vi "change directory permissions.vi"(0 "directory":path=path "C:/Program Files (x86)/National Instruments/RT Images/User Components", 5 "owner":T2={"read"=TRUE, "write"=TRUE, "execute"=TRUE}, 7 "group":T2={"read"=TRUE, "write"=TRUE, "execute"=TRUE}, 9 "others":T2={"read"=TRUE, "write"=TRUE, "execute"=TRUE}, 11 "error in":errorcluster, 12 "action (get)":T1) -> (4 "directory out":path, 6 "permissions":i16 format="%o", 15 "error out":errorcluster)   [LabVIEW 2016]
uses:
  file permissions action.ctl
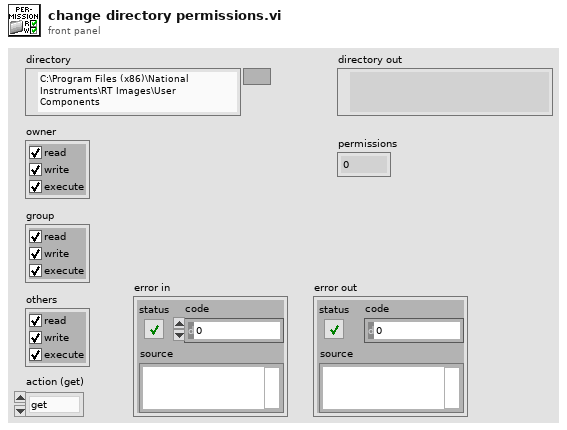
[diagram p1: front panel]
types:
  T1 = typedef "file permissions action.ctl" = enum16{"get", "set", "reset"}
  T2 = cluster{"read":bool, "write":bool, "execute":bool}
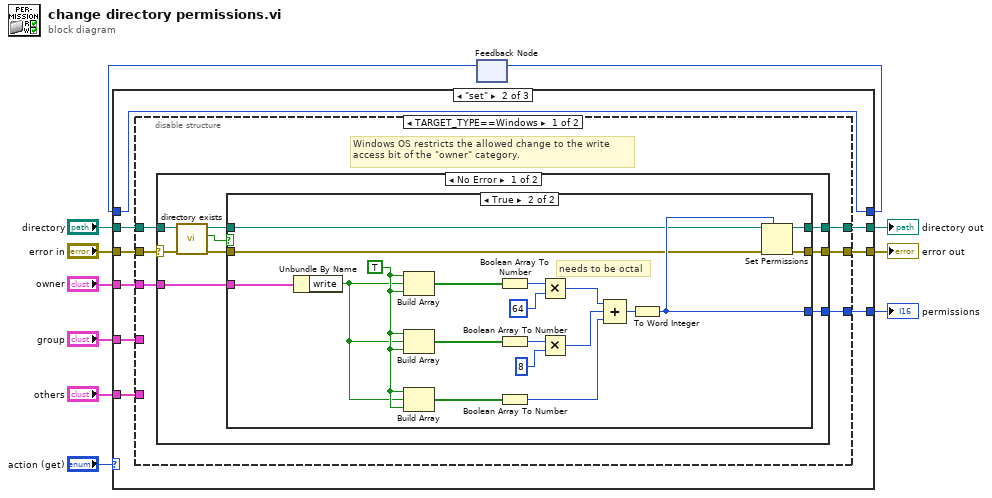
[diagram p0: block diagram]
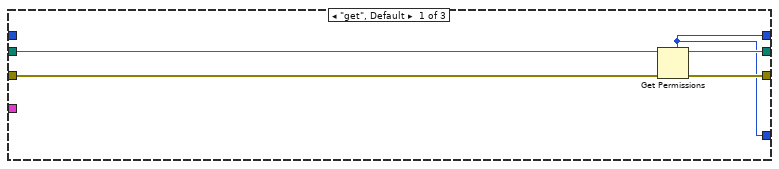
[diagram p2: hidden frame]
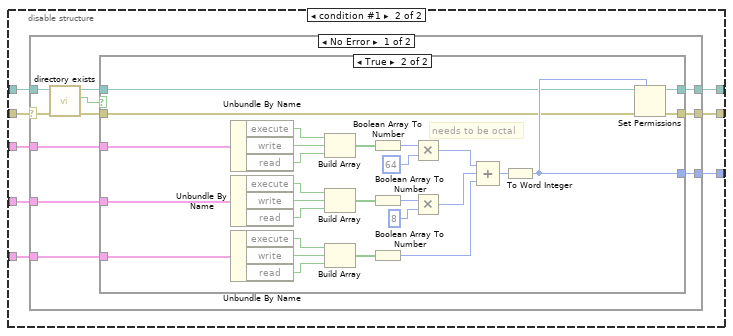
[diagram p5: hidden frame]
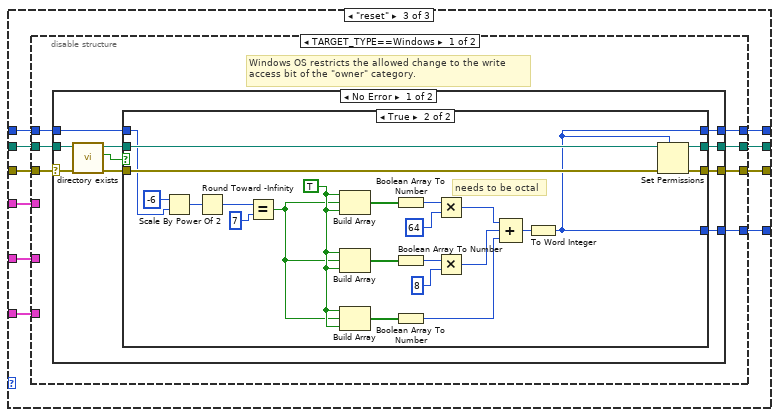
[diagram p8: hidden frame]
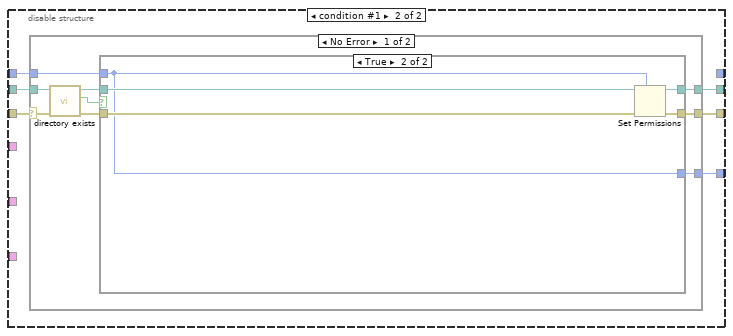
[diagram p11: hidden frame]
diagram:
  n1 = feedback #1() -> (w2:i16)  [unwired: 1 in]
  n2 = case shown="\"set\"" "action (get)" {
    tunnel: "directory" -> [w16 w25 w124]
    tunnel: "error in" -> [w15 w24 w123]
    tunnel: [w12 w17 w117] -> w3
    tunnel: w2 -> [_ w18 w116]
    tunnel: "owner" -> [_ w23 w122]
    tunnel: "group" -> [_ w22 w121]
    tunnel: "others" -> [_ w21 w120]
    tunnel: [w13 w20 w119] -> w4
    tunnel: [w14 w19 w118] -> w5
    tunnel: [w12 w18 w115] -> w1
    frame "get", Default {
      n3 = Get Permissions(8:w15, 11:w16) -> (0:w14:errorcluster, 3:w13:path, 5:w12:i16)  [unwired: 2 out]
    }
    frame "set" {
      n4 = disable-structure shown="TARGET_TYPE==Windows" {
        disable-tunnel: w25 -> [w31 w71]
        disable-tunnel: w24 -> [w26 w66]
        disable-tunnel: w23 -> [w30 w70]
        disable-tunnel: w22 -> [_ w65]
        disable-tunnel: w21 -> [_ w64]
        disable-tunnel: [w28 w68] -> w20
        disable-tunnel: [w27 w67] -> w19
        disable-tunnel: [w29 w69] -> w17
        frame condition #0 (active) {
          # "Windows OS restricts the allowed change to the write\naccess bit of the \"owner\" category."
          n5 = case shown="No Error" w26 {
            selector: w26 -> [w33 w62]
            tunnel: w31 -> [w40 w63]
            tunnel: w30 -> [w39 _]
            tunnel: [w38 _] -> w29
            tunnel: [w35 w63] -> w28
            tunnel: [w34 w62] -> w27
            frame No Error {
              n6 = call "directory exists.vi"("error in"=w33, "directory"=w40) -> ("error out"=w37:errorcluster, "directory present?"=w32:bool, "directory out"=w36:path)  [unwired: 7 in]
              n7 = case shown="True" w32 {
                tunnel: w39 -> [_ w61]
                tunnel: [_ w47] -> w38
                tunnel: w37 -> [w41 w46]
                tunnel: w36 -> [w42 w45]
                tunnel: [w42 w44] -> w35
                tunnel: [w41 w43] -> w34
                frame False {
                  # "#TODO - Add standard file not found error."
                }
                frame True {
                  w51 = TRUE ("read")
                  # "needs to be octal"
                  n8 = Unbundle By Name(w61) -> ("write"=w50:bool)
                  n9 = Build Array(w51, w50, w51) -> (w52:bool[])
                  n10 = Build Array(w51, w50, w51) -> (w49:bool[])
                  n11 = Build Array(w51, w50, w51) -> (w48:bool[])
                  n12 = Boolean Array To Number(Boolean array=w52) -> (number=w54:u16)
                  n13 = Boolean Array To Number(Boolean array=w49) -> (number=w56:u16)
                  n14 = Boolean Array To Number(Boolean array=w48) -> (number=w60:u16)
                  n15 = Multiply(x=w54, y=u16 64) -> (x*y=w58:u16)
                  n16 = Multiply(x=w56, y=u16 8) -> (x*y=w59:u16)
                  n17 = Compound Arithmetic op=ADD(w58, w59, w60) -> (w53:u16)
                  n18 = To Word Integer(number=w53) -> (16bit integer=w47:i16)
                  n19 = Set Permissions(7:w47, 8:w46, 11:w45) -> (0:w43:errorcluster, 3:w44:path)  [unwired: 2 in]
                }
              }
            }
            frame Error {
            }
          }
        }
        frame condition #1 {
          n20 = case shown="No Error" w66 {
            selector: w66 -> [w75 w113]
            tunnel: w71 -> [w82 w114]
            tunnel: w70 -> [w81 _]
            tunnel: [w80 _] -> w69
            tunnel: [w77 w114] -> w68
            tunnel: [w76 w113] -> w67
            tunnel: w65 -> [w73 _]
            tunnel: w64 -> [w72 _]
            frame No Error {
              n21 = call "directory exists.vi"("error in"=w75, "directory"=w82) -> ("error out"=w79:errorcluster, "directory present?"=w74:bool, "directory out"=w78:path)  [unwired: 7 in]
              n22 = case shown="True" w74 {
                tunnel: w81 -> [_ w112]
                tunnel: [_ w99] -> w80
                tunnel: w79 -> [w83 w98]
                tunnel: w78 -> [w84 w97]
                tunnel: [w84 w96] -> w77
                tunnel: [w83 w95] -> w76
                tunnel: w73 -> [_ w94]
                tunnel: w72 -> [_ w93]
                frame False {
                  # "#TODO - Add standard file not found error."
                }
                frame True {
                  # "needs to be octal"
                  n23 = Unbundle By Name(w112) -> ("execute"=w92:bool, "write"=w102:bool, "read"=w91:bool)
                  n24 = Unbundle By Name(w94) -> ("execute"=w90:bool, "write"=w89:bool, "read"=w88:bool)
                  n25 = Unbundle By Name(w93) -> ("execute"=w87:bool, "write"=w86:bool, "read"=w85:bool)
                  n26 = Build Array(w92, w102, w91) -> (w103:bool[])
                  n27 = Build Array(w90, w89, w88) -> (w101:bool[])
                  n28 = Build Array(w87, w86, w85) -> (w100:bool[])
                  n29 = Boolean Array To Number(Boolean array=w103) -> (number=w105:u16)
                  n30 = Boolean Array To Number(Boolean array=w101) -> (number=w107:u16)
                  n31 = Boolean Array To Number(Boolean array=w100) -> (number=w111:u16)
                  n32 = Multiply(x=w105, y=u16 64) -> (x*y=w109:u16)
                  n33 = Multiply(x=w107, y=u16 8) -> (x*y=w110:u16)
                  n34 = Compound Arithmetic op=ADD(w109, w110, w111) -> (w104:u16)
                  n35 = To Word Integer(number=w104) -> (16bit integer=w99:i16)
                  n36 = Set Permissions(7:w99, 8:w98, 11:w97) -> (0:w95:errorcluster, 3:w96:path)  [unwired: 2 in]
                }
              }
            }
            frame Error {
            }
          }
        }
      }
    }
    frame "reset" {
      n37 = disable-structure shown="TARGET_TYPE==Windows" {
        disable-tunnel: w124 -> [w131 w176]
        disable-tunnel: w123 -> [w127 w172]
        disable-tunnel: w122 -> [_ _]
        disable-tunnel: w121 -> [_ _]
        disable-tunnel: w120 -> [_ _]
        disable-tunnel: [w129 w174] -> w119
        disable-tunnel: [w128 w173] -> w118
        disable-tunnel: [w130 w175] -> w117
        disable-tunnel: w116 -> [w126 w171]
        disable-tunnel: [w125 _] -> w115
        frame condition #0 (active) {
          # "Windows OS restricts the allowed change to the write\naccess bit of the \"owner\" category."
          n38 = case shown="No Error" w127 {
            selector: w127 -> [w135 w169]
            tunnel: w131 -> [w141 w170]
            tunnel: [w140 _] -> w130
            tunnel: [w137 w170] -> w129
            tunnel: [w136 w169] -> w128
            tunnel: w126 -> [w133 w168]
            tunnel: [w132 w168] -> w125
            frame No Error {
              n39 = call "directory exists.vi"("error in"=w135, "directory"=w141) -> ("error out"=w139:errorcluster, "directory present?"=w134:bool, "directory out"=w138:path)  [unwired: 7 in]
              n40 = case shown="True" w134 {
                tunnel: [_ w151] -> w140
                tunnel: w139 -> [w143 w155]
                tunnel: w138 -> [w144 w154]
                tunnel: [w144 w153] -> w137
                tunnel: [w143 w152] -> w136
                tunnel: w133 -> [w142 w149]
                tunnel: [w142 w151] -> w132
                frame False {
                  # "#TODO - Add standard file not found error."
                }
                frame True {
                  w158 = TRUE ("read")
                  # "needs to be octal"
                  n41 = Scale By Power Of 2(n=i16 -6, x=w149) -> (x*2^n=w148:i16)
                  n42 = Round Toward -Infinity(1:w148) -> (0:w147:i16)
                  n43 = Equal?(x=w147, y=i16 7) -> (x = y?=w145:bool)
                  n44 = Build Array(w158, w145, w158) -> (w159:bool[])
                  n45 = Build Array(w158, w145, w158) -> (w157:bool[])
                  n46 = Build Array(w158, w145, w158) -> (w156:bool[])
                  n47 = Boolean Array To Number(Boolean array=w159) -> (number=w161:u16)
                  n48 = Boolean Array To Number(Boolean array=w157) -> (number=w163:u16)
                  n49 = Boolean Array To Number(Boolean array=w156) -> (number=w167:u16)
                  n50 = Multiply(x=w161, y=u16 64) -> (x*y=w165:u16)
                  n51 = Multiply(x=w163, y=u16 8) -> (x*y=w166:u16)
                  n52 = Compound Arithmetic op=ADD(w165, w166, w167) -> (w160:u16)
                  n53 = To Word Integer(number=w160) -> (16bit integer=w151:i16)
                  n54 = Set Permissions(7:w151, 8:w155, 11:w154) -> (0:w152:errorcluster, 3:w153:path)  [unwired: 2 in]
                }
              }
            }
            frame Error {
            }
          }
        }
        frame condition #1 {
          n55 = case shown="No Error" w172 {
            selector: w172 -> [w179 w193]
            tunnel: w176 -> [w185 w194]
            tunnel: [w184 _] -> w175
            tunnel: [w181 w194] -> w174
            tunnel: [w180 w193] -> w173
            tunnel: w171 -> [w177 _]
            frame No Error {
              n56 = call "directory exists.vi"("error in"=w179, "directory"=w185) -> ("error out"=w183:errorcluster, "directory present?"=w178:bool, "directory out"=w182:path)  [unwired: 7 in]
              n57 = case shown="True" w178 {
                tunnel: [_ w188] -> w184
                tunnel: w183 -> [w186 w192]
                tunnel: w182 -> [w187 w191]
                tunnel: [w187 w190] -> w181
                tunnel: [w186 w189] -> w180
                tunnel: w177 -> [_ w188]
                frame False {
                  # "#TODO - Add standard file not found error."
                }
                frame True {
                  n58 = Set Permissions(7:w188, 8:w192, 11:w191) -> (0:w189:errorcluster, 3:w190:path)  [unwired: 2 in]
                }
              }
            }
            frame Error {
            }
          }
        }
      }
    }
  }
  "error out" <- w5
  "directory out" <- w4
  "permissions" <- w3
  n59 = feedback-in #1(w1) -> ()
